vi "ReadTriggerArmNode.vi"(8 "Error In":errorcluster, 11 "Multiplexer Node In":refnum<k20>) -> (0 "Error Out":errorcluster, 2 "Trigger Arm Configuration":T1={"Source"=enum."Hold", "Count"=1, "Infinite?"=FALSE} {"Count" min=1 max=99999 step=1}, 3 "Multiplexer Node Out":refnum<k20>)   [LabVIEW 2012]
uses:
  TriggerArmConfiguration.ctl
  driver/Public/Controls/ArmSource.ctl
  <vilib>/xml/NI_XML.lvlib
  driver/Keithley-7001.lvlib
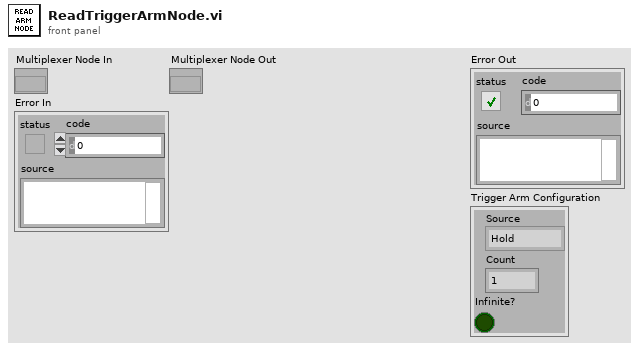
[diagram p1: front panel]
types:
  T1 = typedef "TriggerArmConfiguration.ctl" = cluster{"Source":T2, "Count":u32, "Infinite?":bool}
  T2 = typedef "Keithley-7001.lvlib/ArmSource.ctl" = enum16{"Hold", "Immediate", "Manual", "Bus", "TLink", "External"}
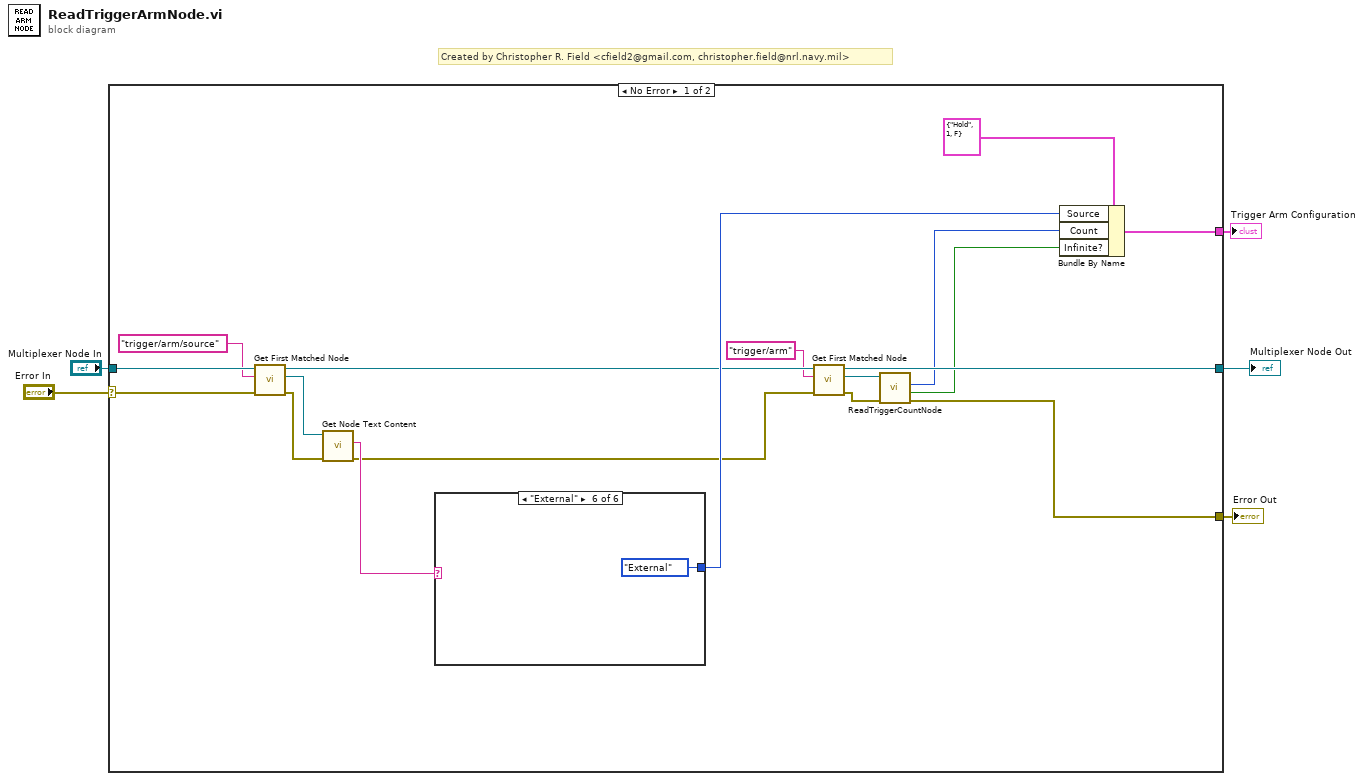
[diagram p0: block diagram]
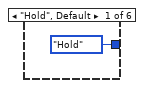
[diagram p2: hidden frame]
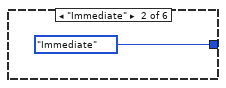
[diagram p3: hidden frame]
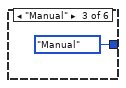
[diagram p4: hidden frame]
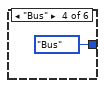
[diagram p5: hidden frame]
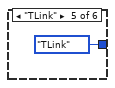
[diagram p6: hidden frame]
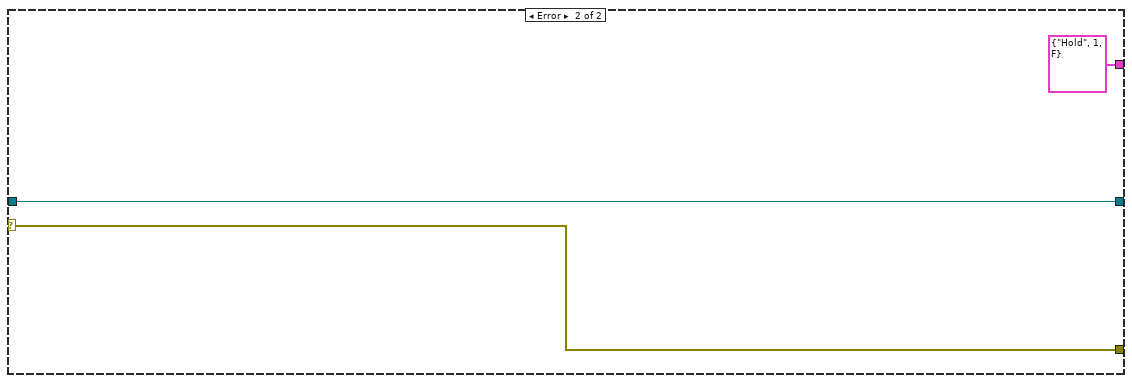
[diagram p7: hidden frame]
diagram:
  # "Created by Christopher R. Field <cfield2@gmail.com, christopher.field@nrl.navy.mil>"
  n1 = case shown="No Error" "Error In" {
    selector: "Error In" -> [w19 w31]
    tunnel: "Multiplexer Node In" -> [w23 w32]
    tunnel: [w10 w31] -> w3
    tunnel: [w9 w32] -> w2
    tunnel: [w6 T1 {"Source"=enum."Hold", "Count"=1, "Infinite?"=FALSE} ("Trigger Arm Configuration")] -> w1
    frame No Error {
      n2 = call <vilib>:"Get First Matched Node.vi"("error in (no error)"=w19, "XPath expression"="trigger/arm/source", "node in"=w23) -> ("error out"=w20:errorcluster, "node result"=w21:refnum<k20>, "node out"=w15:refnum<k20>)  [unwired: 6 in]
      n3 = call <vilib>:"Get Node Text Content.vi"("error in (no error)"=w20, "node in"=w21) -> ("error out"=w12:errorcluster, "node text"=w18:string)  [unwired: 7 in, 1 out]
      n4 = case shown="\"External\"" w18 {
        tunnel: [ArmSource."Hold" ("Arm Source") ArmSource."Immediate" ("Arm Source") ArmSource."Manual" ("Arm Source") ArmSource."Bus" ("Arm Source") ArmSource."TLink" ("Arm Source") ArmSource."External" ("Arm Source")] -> w16
        frame "Hold", Default {
        }
        frame "Immediate" {
        }
        frame "Manual" {
        }
        frame "Bus" {
        }
        frame "TLink" {
        }
        frame "External" {
        }
      }
      n5 = call <vilib>:"Get First Matched Node.vi"("error in (no error)"=w12, "XPath expression"="trigger/arm", "node in"=w15) -> ("error out"=w11:errorcluster, "node result"=w13:refnum<k20>, "node out"=w9:refnum<k20>)  [unwired: 6 in]
      n6 = call "ReadTriggerCountNode.vi"("Error In"=w11, "Trigger Node In"=w13) -> ("Error Out"=w10:errorcluster, "Infinite?"=w7:bool, "Count"=w8:u32)  [unwired: 6 in, 1 out]
      n7 = Bundle By Name(cluster=T1 {"Source"=enum."Hold", "Count"=1, "Infinite?"=FALSE} ("Trigger Arm Configuration"), "Source"=w16, "Count"=w8, "Infinite?"=w7) -> (w6:T1)
    }
    frame Error {
    }
  }
  "Error Out" <- w3
  "Multiplexer Node Out" <- w2
  "Trigger Arm Configuration" <- w1
